vi "init_report.vi"(8 "error in":errorcluster) -> (0 "error out":errorcluster, 2 "appended path":path, 3 "NI_report out":refnum<class "NI_report.lvclass">)   [LabVIEW 2019]
uses:
  <vilib>/Utility/NIReport.llb/NI_report.lvclass
  <vilib>/Utility/NIReport.llb/Report Type.ctl
  FG_save/ae_save_data.ctl
  <vilib>/Utility/NIReport.llb/NI_ReportGenerationCore.lvlib
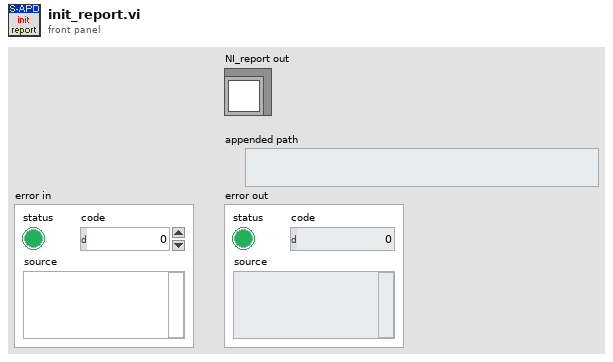
[diagram p1: front panel]
types:
  T1 = typedef "ae_save_data.ctl" = enum16{"create_file", "read", "write", "time", "close_file"}
  T2 = typedef "NI_ReportGenerationCore.lvlib/Report Type.ctl" = enum16{"HTML", "Word", "Excel"}
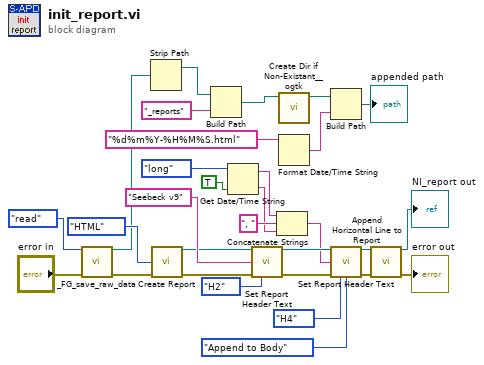
[diagram p0: block diagram]
diagram:
  n1 = call "_FG_save_raw_data.vi"("enum"=ae_save_data."read", "error in"="error in") -> ("path"=w4:path, "error out"=w5:errorcluster)  [unwired: 12 in]
  n2 = Strip Path(path=w4) -> (stripped path=w3:path)  [unwired: 1 out]
  n3 = call <vilib>:"Create Report.vi"("report type"=Report_Type."HTML" ("Report Type"), "error in (no error)"=w5) -> ("report out"=w15:refnum<class "NI_report.lvclass">, "error out"=w14:errorcluster)  [unwired: 12 in]
  n4 = Build Path(base path=w3, name or relative path="_reports") -> (appended path=w2:path)
  n5 = Get Date/Time String(date format (0)=enum16{"short", "long", "abbreviated"}."long" ("format de date (0)"), want seconds? (F)=TRUE ("secondes ? (F)")) -> (date string=w16:string, time string=w8:string)  [unwired: 1 in]
  n6 = call-dynamic "Set Report Header Text.vi"("report in"=w15, "center header text"="Seebeck v9", "error in (no error)"=w14, "HTML header size"=enum16{"H1", "H2", "H3", "H4", "H5", "H6", "H7"}."H2") -> ("report out"=w13:refnum<class "NI_report.lvclass">, "error out"=w11:errorcluster)  [unwired: 10 in]
  n7 = Concatenate Strings(w16, ", " ("chaîne"), w8) -> (w12:string)
  n8 = call <userlib>:"Create Dir if Non-Existant__ogtk.vi"("Directory Path"=w2) -> ("dup Directory Path"=w1:path)  [unwired: 8 in, 2 out]
  n9 = Format Date/Time String(time format string (%c)="%d%m%Y-%H%M%S.html") -> (date/time string=w17:string)  [unwired: 2 in]
  n10 = Build Path(base path=w1, name or relative path=w17) -> (appended path=→"appended path":path)
  n11 = call-dynamic "Set Report Header Text.vi"("report in"=w13, "center header text"=w12, "error in (no error)"=w11, "HTML header size"=enum16{"H1", "H2", "H3", "H4", "H5", "H6", "H7"}."H4", "header placement"=enum16{"Top of Document", "Append to Body"}."Append to Body") -> ("report out"=w10:refnum<class "NI_report.lvclass">, "error out"=w9:errorcluster)  [unwired: 9 in]
  n12 = call-dynamic "Append Horizontal Line to Report.vi"("report in"=w10, "error in (no error)"=w9) -> ("report out"=→"NI_report out":refnum<class "NI_report.lvclass">, "error out"=→"error out":errorcluster)  [unwired: 12 in]
